vi "Xtarget.vi"(1 "Up control in":T1, 2 "Wire in":T2, 8 "Down control in":T1) -> (7 "Wire out":T2)   [LabVIEW 2016]
uses:
  TypeDefs/Circuit Cluster.ctl
  Classes/GateAbst/GateAbst.lvclass
  TypeDefs/Controls.ctl
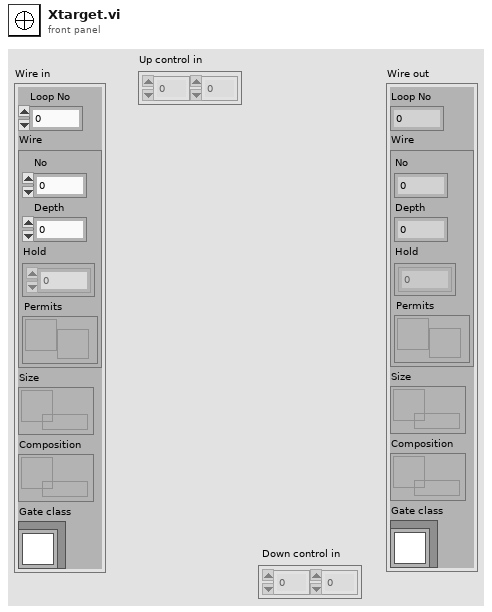
[diagram p1: front panel]
types:
  T1 = typedef "Controls.ctl" = i32[][]
  T2 = typedef "Circuit Cluster.ctl" = cluster{"Loop No":i32, "Wire":cluster{"No":i32, "Depth":i32, "Hold":i32[][], "Permits":refnum<notifier>}, "Size":refnum<queue>, "Composition":refnum<queue>, "Gate class":refnum<class "GateAbst.lvclass">}
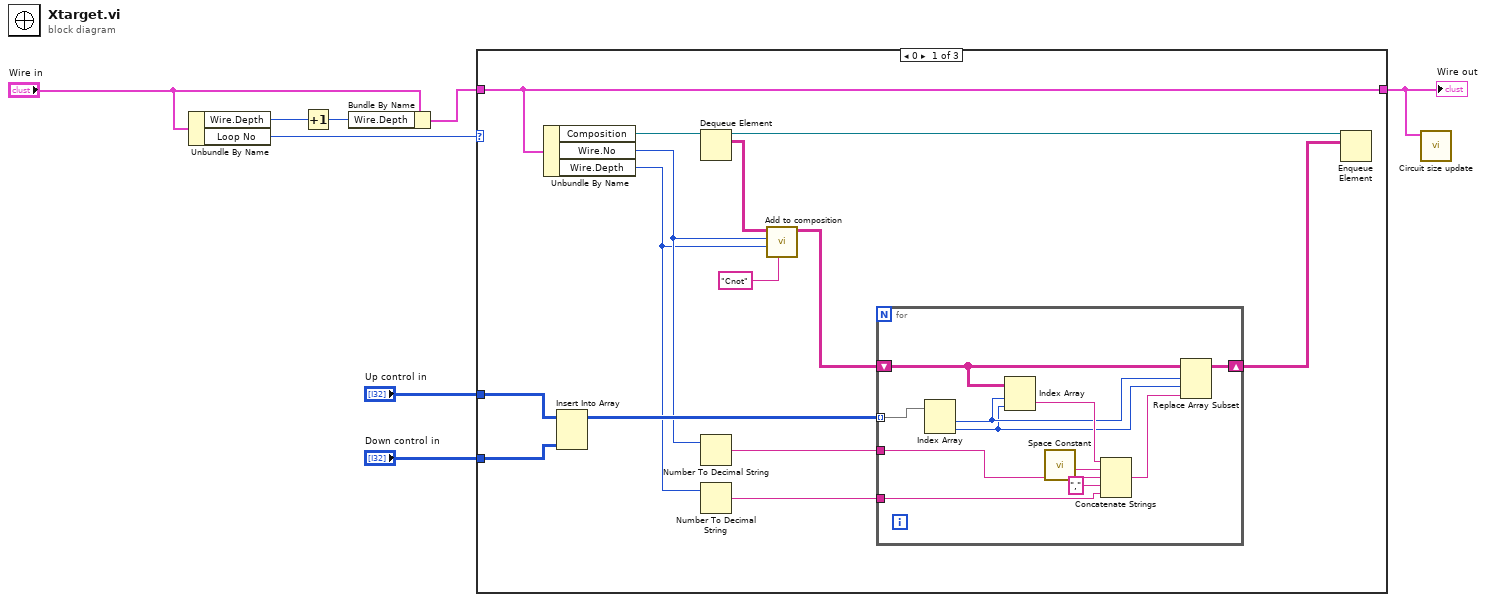
[diagram p0: block diagram]
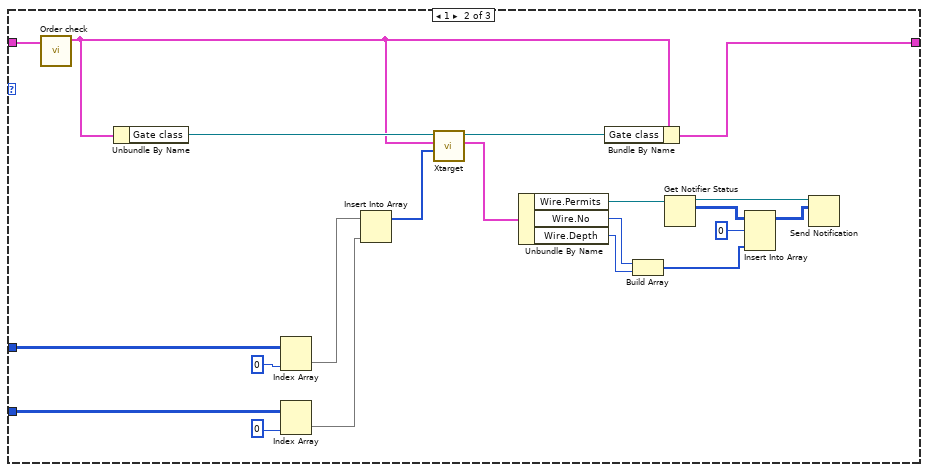
[diagram p2: hidden frame]
diagram:
  n1 = Unbundle By Name("Wire in") -> ("Wire.Depth"=w8:i32, "Loop No"=w1:i32)
  n2 = Increment(x=w8) -> (x+1=w7:i32)
  n3 = Bundle By Name(cluster="Wire in", "Wire.Depth"=w7) -> (w6:T2)
  n4 = case shown="0" w1 {
    tunnel: [w9 w54 w55] -> w2
    tunnel: w6 -> [w9 w34 w55]
    tunnel: "Up control in" -> [w10 w35 _]
    tunnel: "Down control in" -> [w11 w36 _]
    frame 0 {
      n5 = Unbundle By Name(w9) -> ("Composition"=w21:refnum<queue>, "Wire.No"=w17:i32, "Wire.Depth"=w16:i32)
      n6 = Insert Into Array(array=w10, new element=w11) -> (w18:T1)  [unwired: 2 in]
      n7 = Dequeue Element(queue=w21) -> (queue out=w22:refnum<queue>, element=w20:string[][])  [unwired: 2 in, 2 out]
      n8 = Number To Decimal String(number=w17) -> (decimal integer string=w15:string)  [unwired: 1 in]
      n9 = Number To Decimal String(number=w16) -> (decimal integer string=w14:string)  [unwired: 1 in]
      n10 = call "Add to composition.vi"("Gate name"="Cnot", "Wire depth"=w16, "Wire No"=w17, "Composition in"=w20) -> ("Composition out"=w13:string[][])  [unwired: 7 in]
      n11 = for {
        tunnel: w18 -> [w33] mode=indexing
        tunnel: w15 -> [w30]
        tunnel: w14 -> [w28]
        shift-right: [w24] -> w12
        shift-left: w13 -> [w23]
        n12 = Index Array(array=w33) -> (element #1=w27:i32, element #2=w26:i32)  [unwired: 2 in]
        n13 = Index Array(array=w23, index (row)=w27, index (col)=w26) -> (element=w32:string)
        n14 = call <vilib>:"Space Constant.vi"() -> ("String"=w31:string)
        n15 = Concatenate Strings(w32, w31, w30, "," ("string"), w28) -> (w25:string)
        n16 = Replace Array Subset(array=w23, new element=w25, index (row)=w27, index (col)=w26) -> (w24:string[][])
      }
      n17 = Enqueue Element(queue=w22, element=w12) -> ()  [unwired: 2 in, 3 out]
    }
    frame 1 {
      n18 = call "Order check.vi"("Wire in in"=w34) -> ("Wire out"=w43:T2)  [unwired: 10 in]
      n19 = Unbundle By Name(w43) -> ("Gate class"=w52:refnum<class "GateAbst.lvclass">)
      n20 = Index Array(array=w35, index (col)=0 ("disabled index (col)")) -> (element=w48:i32[])  [unwired: 1 in]
      n21 = Index Array(array=w36, index (col)=0 ("disabled index (col)")) -> (element=w47:i32[])  [unwired: 1 in]
      n22 = Insert Into Array(array=w48, new element=w47) -> (w46:i32[])  [unwired: 1 in]
      n23 = call-dynamic "Xtarget.vi"("Controls"=w46, "Target in"=w43, "GateAbst in"=w52) -> ("Target out"=w51:T2, "GateAbst out"=w53:refnum<class "GateAbst.lvclass">)  [unwired: 6 in, 1 out]
      n24 = Unbundle By Name(w51) -> ("Wire.Permits"=w42:refnum<notifier>, "Wire.No"=w45:i32, "Wire.Depth"=w44:i32)
      n25 = Bundle By Name(cluster=w43, "Gate class"=w53) -> (w54:T2)
      n26 = Build Array(w45, w44) -> (w39:i32[])
      n27 = Get Notifier Status(notifier=w42) -> (notifier out=w38:refnum<notifier>, current notification=w41:i32[][])  [unwired: 1 in, 3 out]
      n28 = Insert Into Array(array=w41, index (row)=0, new element=w39) -> (w37:i32[][])  [unwired: 1 in]
      n29 = Send Notification(notification=w37, notifier=w38) -> ()  [unwired: 1 in, 2 out]
    }
    frame Default {
    }
  }
  "Wire out" <- w2
  n30 = call "Circuit size update.vi"("Wire in"=w2) -> ()  [unwired: 11 in]
